vi "斐波那契数列.vi"(1 "数值":u32) -> (0 "数值 2":u32)   [LabVIEW 2023]
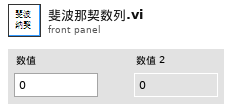
[diagram p1: front panel]
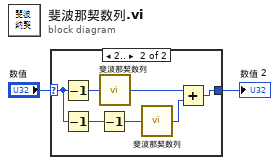
[diagram p0: block diagram]
diagram:
  n1 = case shown="2.." "数值" {
    selector: "数值" -> [w3 w9]
    tunnel: [w3 w4] -> w1
    frame ..1, Default {
    }
    frame 2.. {
      n2 = Decrement(x=w9) -> (x-1=w10:u32)
      n3 = Decrement(x=w9) -> (x-1=w8:u32)
      n4 = Decrement(x=w8) -> (x-1=w7:u32)
      n5 = call "斐波那契数列.vi"("数值"=w10) -> ("数值 2"=w6:u32)
      n6 = call "斐波那契数列.vi"("数值"=w7) -> ("数值 2"=w5:u32)
      n7 = Add(x=w6, y=w5) -> (x+y=w4:u32)
    }
  }
  "数值 2" <- w1
